vi "GetFirstCharacterInformation.vi"(8 "error in (no error)":errorcluster, 11 "EAN-13 In":refnum<class "EAN-13.lvclass">) -> (0 "error out":errorcluster, 2 "Text Information":T1, 3 "EAN-13 out":refnum<class "EAN-13.lvclass">)   [LabVIEW 2013, in "BarCodes.lvlib" / "EAN-13.lvclass"]
uses:
  EAN-13.lvclass
  BarCode/TextPosition.ctl
  BarCodes.lvlib
  BarCode/BarCode.lvclass
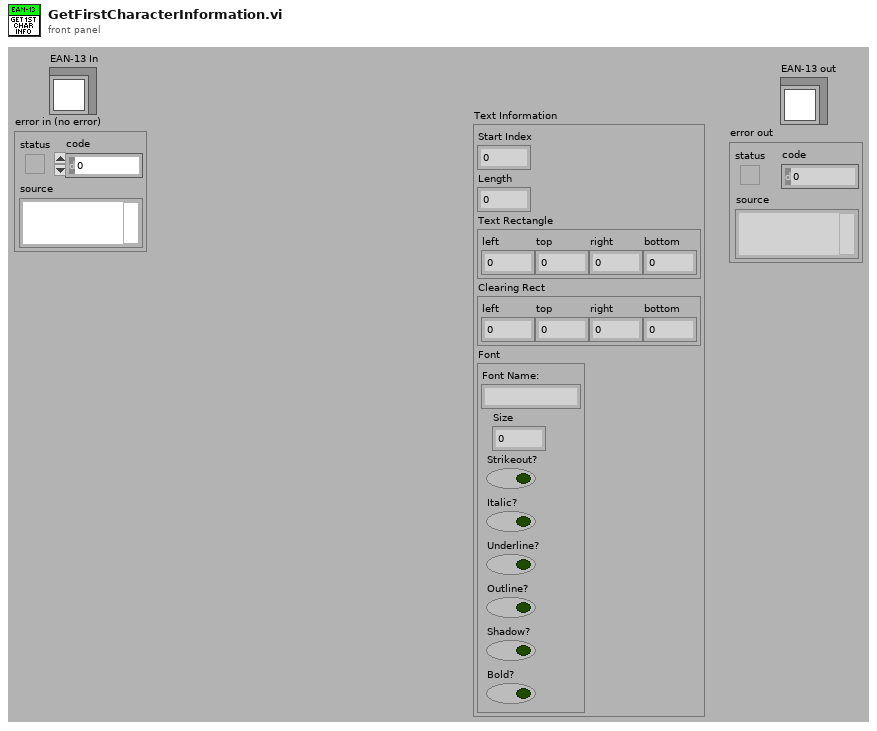
[diagram p1: front panel]
types:
  T1 = typedef "BarCodes.lvlib/BarCode.lvclass/TextPosition.ctl" = cluster{"Start Index":u8, "Length":u8, "Text Rectangle":cluster{"left":i16, "top":i16, "right":i16, "bottom":i16}, "Clearing Rect":cluster{"left":i16, "top":i16, "right":i16, "bottom":i16}, "Font":cluster{"Font Name:":string, "Size":i16, "Strikeout?":bool, "Italic?":bool, "Underline?":bool, "Outline?":bool, "Shadow?":bool, "Bold?":bool}}
  T2 = cluster{"left":i32, "top":i16, "right":i16, "bottom":i16}
  T3 = cluster{"left":i16, "top":i16, "right":i16, "bottom":i16}
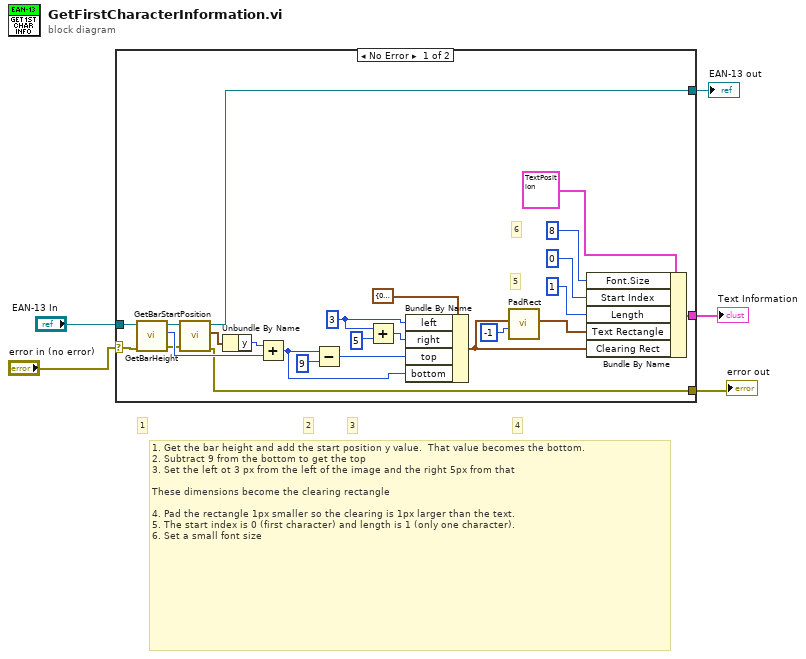
[diagram p0: block diagram]
diagram:
  # "4"
  # "3"
  # "2"
  # "1"
  # "1. Get the bar height and add the start position y value.  That value becomes the bottom.\n2. Subtract 9 from the bottom to get the top\n3. Set the left ot 3 px from the left of the image and the right 5px from that\n\nThese dimensions become the clearing rectangle\n\n4. Pad the rectangle 1px smaller so the clearing is 1px larger than the text.\n5. The start index is 0 (first character) and length is 1 (only one character).\n6. Set a small font size"
  n1 = case shown="No Error" "error in (no error)" {
    selector: "error in (no error)" -> [w6 w30]
    tunnel: [w29 _] -> w5
    tunnel: "EAN-13 In" -> [w17 w31]
    tunnel: [w14 w31] -> w3
    tunnel: [w7 w30] -> w2
    frame No Error {
      w21 = i16 3 ("y")
      # "6"
      # "5"
      n2 = call-dynamic "GetBarHeight.vi"("error in (no error)"=w6, "EAN-13 in"=w17) -> ("error out"=w8:errorcluster, "Bar Height"=w16:u8, "EAN-13 out"=w15:refnum<class "EAN-13.lvclass">)  [unwired: 7 in]
      n3 = call-dynamic "GetBarStartPosition.vi"("error in (no error)"=w8, "EAN-13 in"=w15) -> ("error out"=w7:errorcluster, "Start Position"=w13:cluster{"x":i16, "y":i16}, "EAN-13 out"=w14:refnum<class "EAN-13.lvclass">)  [unwired: 7 in]
      n4 = Unbundle By Name(w13) -> ("y"=w12:i16)
      n5 = Add(x=w12, y=w16) -> (x+y=w9:i16)
      n6 = Subtract(x=w9, y=i16 9) -> (x-y=w20:i16)
      n7 = Add(x=w21, y=i16 5) -> (x+y=w19:i16)
      n8 = Bundle By Name(cluster=T2 {"left"=0, "top"=0, "right"=0, "bottom"=0} ("Text Rectagle"), "left"=w21, "right"=w19, "top"=w20, "bottom"=w9) -> (w10:T2)
      n9 = call "PadRect.vi"("Padding"=i8 -1, "Rectagle"=w10) -> ("Padded Rectangle"=w11:T3)  [unwired: 9 in]
      n10 = Bundle By Name(cluster=T1 {"Start Index"=0, "Length"=0, "Text Rectangle"={"left"=0, "top"=0, "right"=0, "bottom"=0}, "Clearing Rect"={"left"=0, "top"=0, "right"=0, "bottom"=0}, "Font"={"Font Name:"="Application Font", "Size"=12, "Strikeout?"=FALSE, "Italic?"=FALSE, "Underline?"=FALSE, "Outline?"=FALSE, "Shadow?"=FALSE, "Bold?"=FALSE}} ("Text Position 2"), "Font.Size"=i16 8, "Start Index"=u8 0, "Length"=u8 1 ("End Index"), "Text Rectangle"=w11, "Clearing Rect"=w10) -> (w29:T1)
    }
    frame Error {
    }
  }
  "Text Information" <- w5
  "EAN-13 out" <- w3
  "error out" <- w2
